vi "is connection upgraded.vi"(11 "data in":string) -> (3 "upgrade response":bool)   [LabVIEW 2016, in "websocket client.lvclass"]
uses:
  websocket client.lvclass
  <vilib>/Utility/error.llb/whitespace.ctl
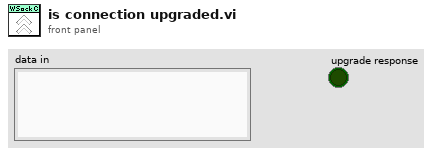
[diagram p1: front panel]
types:
  T1 = typedef "whitespace.ctl" = u16
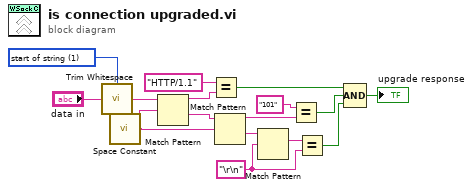
[diagram p0: block diagram]
diagram:
  w1 = T1 1 items=["both", "start of string", "end of string"] ("location (both)")
  w6 = "\r\n"
  n1 = call <vilib>:"Trim Whitespace.vi"("string"="data in", "location (both)"=w1) -> ("trimmed string"=w2:string)
  n2 = call <vilib>:"Space Constant.vi"() -> ("String"=w3:string)
  n3 = Match Pattern(string=w2, regular expression=w3) -> (before substring=w9:string, after substring=w5:string)  [unwired: 1 in, 2 out]
  n4 = Equal?(x="HTTP/1.1", y=w9) -> (x = y?=w14:bool)
  n5 = Match Pattern(string=w5, regular expression=w3) -> (before substring=w12:string, after substring=w4:string)  [unwired: 1 in, 2 out]
  n6 = Match Pattern(string=w4, regular expression=w6) -> (match substring=w7:string)  [unwired: 1 in, 3 out]
  n7 = Equal?(x="101", y=w12) -> (x = y?=w13:bool)
  n8 = Equal?(x=w7, y=w6) -> (x = y?=w15:bool)
  n9 = Compound Arithmetic op=AND(w14, w13, w15) -> (→"upgrade response":bool)
